vi "G4BaseTemplate_Singleton_6x8x6_CleanUp.vi"(5 "Error In":errorcluster) -> (19 "Error Out":errorcluster)   [LabVIEW 2020, in "G4BaseTemplate_Singleton_6x8x6.lvclass"]
uses:
  <resource>/Framework/Providers/Open_GDS/ClassProviders/Provider_EndevoGOOP400/Templates/G4BaseTemplate_Singleton_6x8x6/G4BaseTemplate_Singleton_6x8x6.lvclass
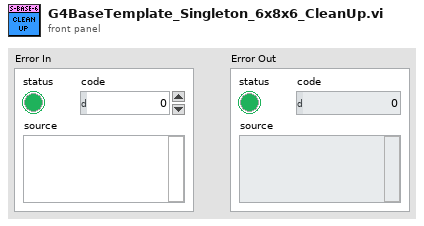
[diagram p1: front panel]
types:
  T1 = typedef "G4BaseTemplate_Singleton_6x8x6.lvclass/ObjectAttributes.ctl" = cluster{"Attribute1":dbl}
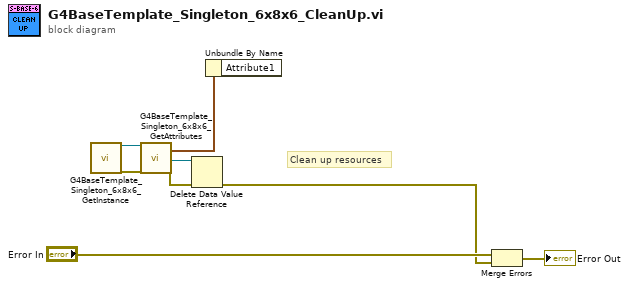
[diagram p0: block diagram]
diagram:
  # "Clean up resources"
  n1 = call <resource>:"G4BaseTemplate_Singleton_6x8x6_GetInstance.vi"() -> ("reference out"=w5:refnum<class "G4BaseTemplate_Singleton_6x8x6.lvclass">, "Error Out"=w6:errorcluster)  [unwired: 15 in, 3 out]
  n2 = call <resource>:"G4BaseTemplate_Singleton_6x8x6_GetAttributes.vi"("reference in"=w5, "Error In"=w6) -> ("Data"=w7:T1, "DataRef"=w3:refnum<data-value>, "Error Out"=w4:errorcluster)  [unwired: 14 in, 1 out]
  n3 = Delete Data Value Reference(data value reference=w3, error in=w4) -> (error out=w1:errorcluster)  [unwired: 1 out]
  n4 = Unbundle By Name(w7) -> ()  [unwired: 1 out]
  n5 = Merge Errors("Error In", w1) -> (→"Error Out":errorcluster)
